vi "TSLIN_Queue_Init.vi"(8 "error in (no error)":errorcluster caption="错误输入（无错误）", 10 "receiver":string, 11 "Channels used":u16) -> (0 "error out":errorcluster caption="错误输出")   [LabVIEW 2014]
uses:
  <vilib>/Utility/miscctls.llb/LVPointTypeDef.ctl
panel:
  out "Initializing...":u8(slide) scale=0.0..100.0
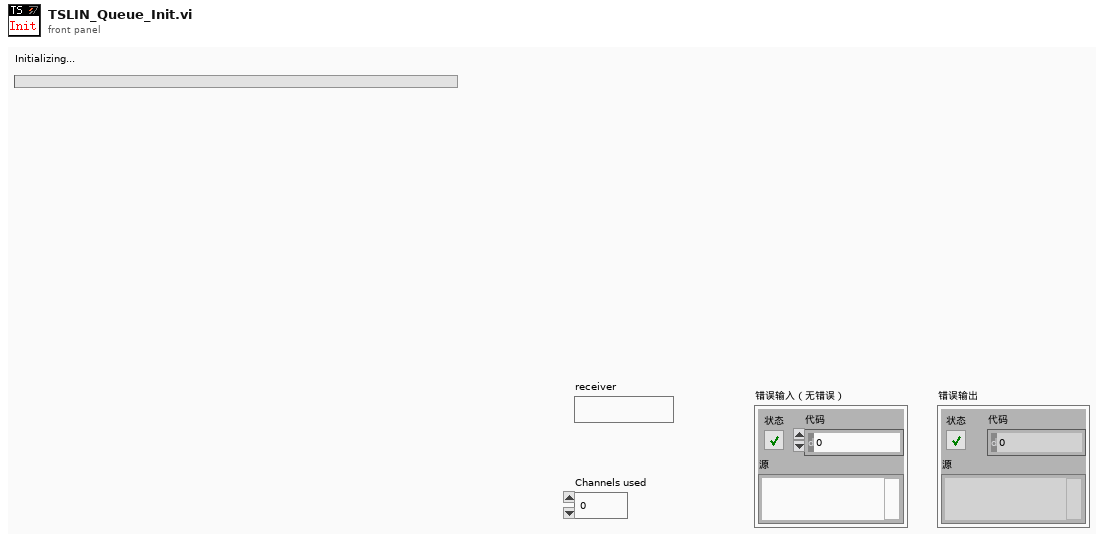
[diagram p1: front panel]
types:
  T1 = typedef "LVPointTypeDef.ctl" = cluster{"Horizontal":i16, "Vertical":i16}
  T2 = cluster{"Sender":string, "receiver":string, "message":string, "data":variant}
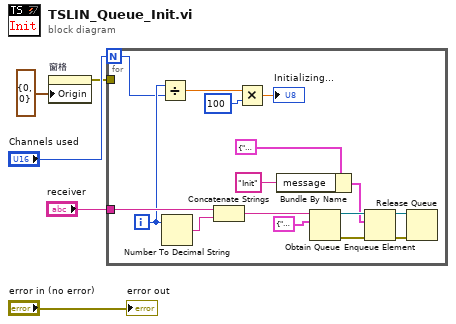
[diagram p0: block diagram]
diagram:
  n1 = property on="窗格" class="Pane"("Origin"=T1 {"Horizontal"=0, "Vertical"=0} ("原点")) -> (error out=w2:errorcluster)  [unwired: 2 in, 1 out]
  n2 = for {
    N: "Channels used" -> [w9]
    tunnel: "receiver" -> [w16]
    tunnel: w2 -> [_]
    i -> [w10]
    n3 = Divide(x=w10, y=w9) -> (x/y=w13:dbl)
    n4 = Number To Decimal String(number=w10) -> (decimal integer string=w17:string)  [unwired: 1 in]
    n5 = Concatenate Strings(w16, w17) -> (w15:string)
    n6 = Multiply(x=w13, y=u8 100) -> (x*y=→"Initializing...":dbl)
    n7 = Bundle By Name(cluster=T2 {"Sender"="", "receiver"="", "message"="Quit", "data"=variant} ("元素"), "message"="Init") -> (w7:T2)
    n8 = Obtain Queue(name (unnamed)=w15, element data type=T2 {"Sender"="", "receiver"="", "message"="", "data"=variant} ("Communication message")) -> (queue out=w21:refnum<queue>, error out=w19:errorcluster)  [unwired: 3 in, 1 out]
    n9 = Enqueue Element(queue=w21, element=w7, error in (no error)=w19) -> (queue out=w20:refnum<queue>, error out=w18:errorcluster)  [unwired: 1 in, 1 out]
    n10 = Release Queue(queue=w20, error in (no error)=w18) -> ()  [unwired: 1 in, 3 out]
  }
  "error out" <- "error in (no error)"
